vi "FPGA Close.vi"(8 "Error In":errorcluster, 11 "FPGA VI Reference In":refnum<k20>) -> (0 "Error Out":errorcluster)   [LabVIEW 2018]
uses:
  <vilib>/FPGAPlugInAG/PXIe-5840/niLvFpga_Close_PXIe-5840.vi
  <vilib>/rvi/interface/nirviCloseFPGA/nirviCloseFPGA.xnode
  Program Files (x86)/National Instruments/LabVIEW 2018/instr.lib/niVST/FPGA/Templates/FPGA Bitfiles/niVSTFPGA_UART.lvbitx
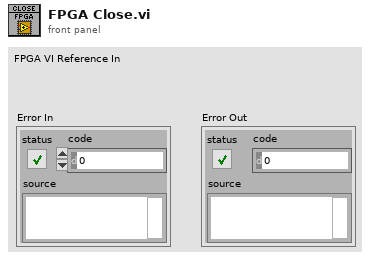
[diagram p1: front panel]
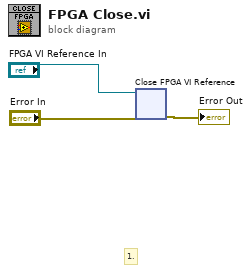
[diagram p0: block diagram]
diagram:
  # "1."
  n1 = xnode "Close FPGA VI Reference"("FPGA VI Reference In"="FPGA VI Reference In", "error in"="Error In") -> ("error out"=→"Error Out":errorcluster)
